vi "Run FGV Tests for Double.vi"(2 "DELETE VI Reference":refnum<vi>, 3 "GET VI Reference":refnum<vi>, 4 "PUT VI Reference":refnum<vi>) -> (0 "Reason":string, 1 "Success":bool)   [LabVIEW 2013]
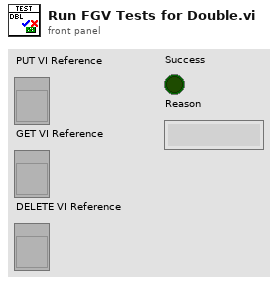
[diagram p1: front panel]
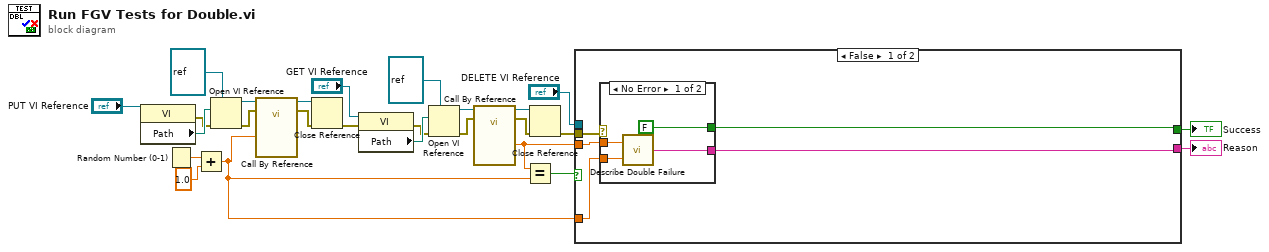
[diagram p0: block diagram]
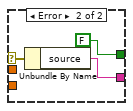
[diagram p2: hidden frame]
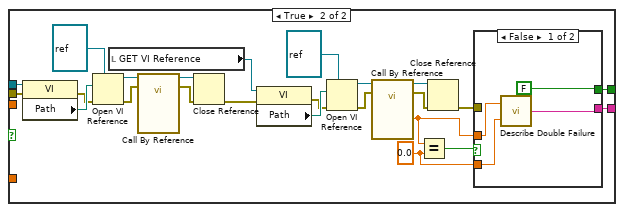
[diagram p3: hidden frame]
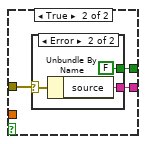
[diagram p4: hidden frame]
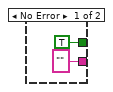
[diagram p5: hidden frame]
diagram:
  n1 = property class="VI"(reference="PUT VI Reference") -> (error out=w3:errorcluster, "Path"=w17:path)  [unwired: 1 in, 1 out]
  n2 = Random Number (0-1)() -> (number: 0 to 1=w11:dbl)
  n3 = Add(x=w11, y=1.0) -> (x+y=w6:dbl)
  n4 = Open VI Reference(type specifier VI Refnum (for type only)=refnum<vi> refnum, vi path=w17, error in (no error)=w3) -> (vi reference=w16:refnum<vi>, error out=w15:errorcluster)  [unwired: 3 in]
  n5 = call-by-ref "?"(reference=w16, error in=w15, "Maximum Input Voltage"=w6) -> (reference out=w14:refnum<vi>, error out=w13:errorcluster)
  n6 = Close Reference(reference=w14, error in (no error)=w13) -> (error out=w9:errorcluster)
  n7 = property class="VI"(reference="GET VI Reference", error in=w9) -> (error out=w4:errorcluster, "Path"=w22:path)  [unwired: 1 out]
  n8 = Open VI Reference(type specifier VI Refnum (for type only)=refnum<vi> refnum, vi path=w22, error in (no error)=w4) -> (vi reference=w23:refnum<vi>, error out=w24:errorcluster)  [unwired: 3 in]
  n9 = call-by-ref "?"(reference=w23, error in=w24) -> (reference out=w25:refnum<vi>, error out=w26:errorcluster, "Calibration Sample Rate"=w5:dbl)
  n10 = Equal?(x=w5, y=w6) -> (x = y?=w7:bool)
  n11 = Close Reference(reference=w25, error in (no error)=w26) -> (error out=w8:errorcluster)
  n12 = case shown="False" w7 {
    tunnel: "DELETE VI Reference" -> [_ w56]
    tunnel: w8 -> [w27 w55]
    tunnel: w6 -> [w30 _]
    tunnel: w5 -> [w31 _]
    tunnel: [w29 w40] -> w2
    tunnel: [w28 w39] -> w1
    frame False {
      n13 = case shown="No Error" w27 {
        selector: w27 -> [_ w38]
        tunnel: w31 -> [w35 _]
        tunnel: w30 -> [w34 _]
        tunnel: [FALSE FALSE] -> w29
        tunnel: [w32 w36] -> w28
        frame No Error {
          n14 = call "Describe Double Failure.vi"("Expected"=w34, "Got"=w35) -> ("Failure Description"=w32:string)
        }
        frame Error {
          n15 = Unbundle By Name(w38) -> ("source"=w36:string)
        }
      }
    }
    frame True {
      w41 = 0.0 ("y")
      n16 = property class="VI"(reference=w56, error in=w55) -> (error out=w45:errorcluster, "Path"=w58:path)  [unwired: 1 out]
      n17 = Open VI Reference(type specifier VI Refnum (for type only)=refnum<vi> refnum, vi path=w58, error in (no error)=w45) -> (vi reference=w59:refnum<vi>, error out=w60:errorcluster)  [unwired: 3 in]
      n18 = local read "GET VI Reference"() -> (w43:refnum<vi>)
      n19 = call-by-ref "?"(reference=w59, error in=w60) -> (reference out=w61:refnum<vi>, error out=w62:errorcluster)  [unwired: 1 in]
      n20 = Close Reference(reference=w61, error in (no error)=w62) -> (error out=w48:errorcluster)
      n21 = property class="VI"(reference=w43, error in=w48) -> (error out=w46:errorcluster, "Path"=w50:path)  [unwired: 1 out]
      n22 = Open VI Reference(type specifier VI Refnum (for type only)=refnum<vi> refnum, vi path=w50, error in (no error)=w46) -> (vi reference=w51:refnum<vi>, error out=w52:errorcluster)  [unwired: 3 in]
      n23 = call-by-ref "?"(reference=w51, error in=w52) -> (reference out=w53:refnum<vi>, error out=w54:errorcluster, "Calibration Sample Rate"=w42:dbl)
      n24 = Equal?(x=w42, y=w41) -> (x = y?=w47:bool)
      n25 = Close Reference(reference=w53, error in (no error)=w54) -> (error out=w44:errorcluster)
      n26 = case shown="False" w47 {
        tunnel: w44 -> [_ w69]
        tunnel: w42 -> [w66 _]
        tunnel: w41 -> [w65 _]
        tunnel: [FALSE w68] -> w40
        tunnel: [w63 w67] -> w39
        frame False {
          n27 = call "Describe Double Failure.vi"("Expected"=w65, "Got"=w66) -> ("Failure Description"=w63:string)
        }
        frame True {
          n28 = case shown="Error" w69 {
            selector: w69 -> [_ w74]
            tunnel: [TRUE FALSE] -> w68
            tunnel: ["" ("source") w72] -> w67
            frame No Error {
            }
            frame Error {
              n29 = Unbundle By Name(w74) -> ("source"=w72:string)
            }
          }
        }
      }
    }
  }
  "Success" <- w2
  "Reason" <- w1
